vi "Reprocess fit.vi"() -> ()   [LabVIEW 2016]
uses:
  Utilities/Fit/Multi-peak Parameters.ctl
  Utilities/Fit/Peak Parameters.ctl
panel:
  out "XY Graph":cluster{dbl[], dbl[]}(graph)
  out "Fit parameters out":T1={"Function"=enum."Gauss", "Window width"=nan, "Initial guess"={"Amplitude"=1000.0, "Center"=694.3, "Width"=0.4}} {"Initial guess"."Width" format="%#_gnm"; "Initial guess"."Center" format="%#_gnm"; "Window width" format="%#_6gnm"}
  out "Temperature":dbl
  out "Spectral Waveform":cluster{"Array":dbl[], "Array":dbl[]}[](graph)
  in  "Only once":bool
  in  "Fit parameters":T1={"Function"=enum."Lorentz", "Window width"=1.0, "Initial guess"={"Amplitude"=1000.0, "Center"=694.3, "Width"=0.4}} {"Initial guess"."Width" format="%#_gnm"; "Initial guess"."Center" format="%#_gnm"; "Window width" format="%#_6gnm"}
  in  "Channel T":string="Neocera 21 (15) A"
  in  "Channel Wavelength":string="Wavelengths"
  in  "New  file":path
  in  "Spectrum file":path
  in  "Channel":string="Avg Amplitude"
  in  "Group":string="p"
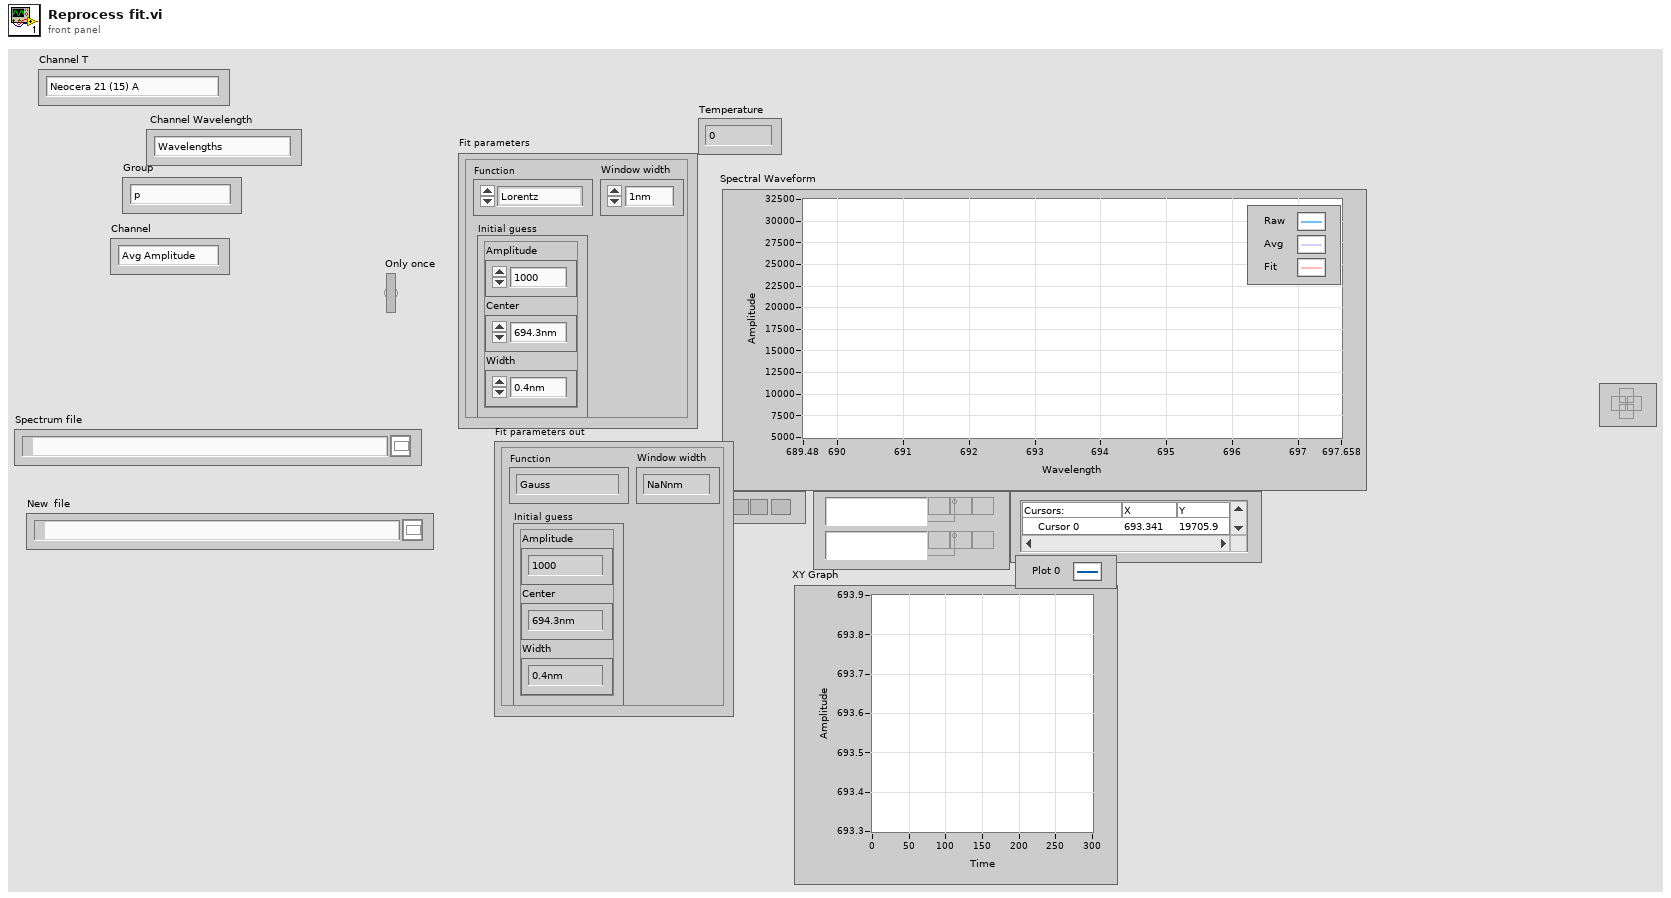
[diagram p1: front panel]
types:
  T1 = typedef "Multi-peak Parameters.ctl" = cluster{"Function":enum16{"Gauss", "Lorentz"}, "Window width":dbl, "Initial guess":T2}
  T2 = typedef "Peak Parameters.ctl" = cluster{"Amplitude":dbl, "Center":dbl, "Width":dbl}
  T3 = enum16{"open", "open or create", "create or replace", "create", "open (read-only)"}
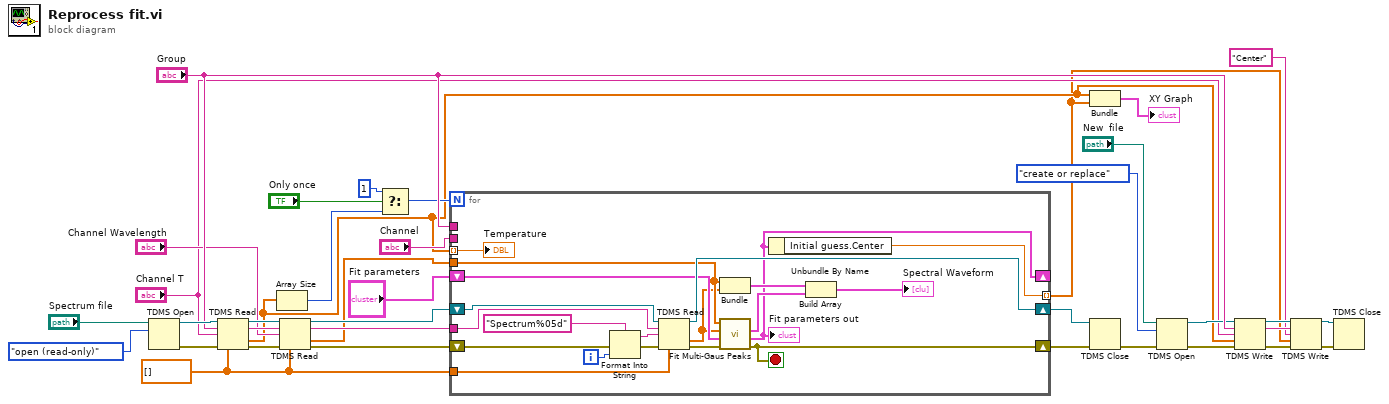
[diagram p0: block diagram]
diagram:
  w22 = dbl[] []
  n1 = TDMS Open(10:T3."open (read-only)" ("operation (0:open)"), 11:"Spectrum file") -> (0:w30:errorcluster, 3:w31:refnum<k34>)  [unwired: 5 in]
  n2 = TDMS Read(0:w31, 5:"Group", 7:"Channel T", 11:w30, 12:w22) -> (4:w27:refnum<k34>, 6:w24:string, 10:w4:dbl[], 15:w29:errorcluster)  [unwired: 3 in, 2 out]
  n3 = Array Size(array=w4) -> (size(s)=w19:i32)
  n4 = TDMS Read(0:w27, 5:w24, 7:"Channel Wavelength", 11:w29, 12:w22) -> (4:w26:refnum<k34>, 6:w23:string, 10:w14:dbl[], 15:w28:errorcluster)  [unwired: 3 in, 2 out]
  n5 = Select(t=1, s="Only once", f=w19) -> (s? t:f=w16:i32)
  n6 = for {
    N: w16 -> [_]
    tunnel: w22 -> [w55]
    tunnel: "Group" -> [_]
    tunnel: "Channel" -> [_]
    shift-right: [w46] -> w37
    shift-left: w28 -> [w51]
    shift-right: [w57] -> w36
    shift-left: w26 -> [w56]
    tunnel: w23 -> [w54]
    shift-right: [w39] -> _
    shift-left: "Fit parameters" -> [w48]
    tunnel: w14 -> [w44]
    tunnel: w4 -> [w40] mode=indexing
    tunnel: [w38] -> w3 mode=indexing
    i -> [w52]
    stop <- w46 stop-if-true
    n7 = Format Into String(format string="Spectrum%05d", error in=w51, w52) -> (resulting string=w49:string, error out=w50:errorcluster)  [unwired: 1 in]
    n8 = TDMS Read(0:w56, 5:w54, 7:w49, 11:w50, 12:w55) -> (4:w57:refnum<k34>, 10:w43:dbl[], 15:w47:errorcluster)  [unwired: 3 in, 3 out]
    n9 = Bundle(w44, w43) -> (w41:cluster{dbl[], dbl[]})  [unwired: 1 in]
    n10 = call "Fit Multi-Gaus Peaks.vi"("Error In"=w47, "Fit parameters"=w48, "Y"=w43, "X"=w44) -> ("Error Out"=w46:errorcluster, "Fit parameters out"=w39:T1, "Fit plot"=w45:cluster{"Array":dbl[], "Array":dbl[]})  [unwired: 5 in]
    "Fit parameters out" <- w39
    n11 = Unbundle By Name(w39) -> ("Initial guess.Center"=w38:dbl)
    n12 = Build Array(w41, w45) -> (→"Spectral Waveform":cluster{"Array":dbl[], "Array":dbl[]}[])
    "Temperature" <- w40
  }
  n13 = Bundle(w4, w3) -> (→"XY Graph":cluster{dbl[], dbl[]})  [unwired: 1 in]
  n14 = TDMS Close(8:w37, 11:w36) -> (0:w1:errorcluster)  [unwired: 1 out]
  n15 = TDMS Open(8:w1, 10:T3."create or replace" ("operation (0:open)"), 11:"New  file") -> (0:w11:errorcluster, 3:w12:refnum<k34>)  [unwired: 4 in]
  n16 = TDMS Write(0:w12, 5:"Group", 7:"Channel T", 9:w4, 11:w11) -> (4:w10:refnum<k34>, 6:w6:string, 15:w8:errorcluster)  [unwired: 1 in, 1 out]
  n17 = TDMS Write(0:w10, 5:w6, 7:"Center" ("Channel"), 9:w3, 11:w8) -> (4:w9:refnum<k34>, 15:w7:errorcluster)  [unwired: 1 in, 2 out]
  n18 = TDMS Close(8:w7, 11:w9) -> ()  [unwired: 2 out]
